vi "Set Stage Speed.vi"(8 "error in (no error)":errorcluster, 9 "Y Axis":u16, 10 "X Axis":u16, 11 "2-Axis Stage in":refnum<class "XY Stage Controller.lvclass">) -> (0 "error out":errorcluster, 3 "2-Axis Stage out":refnum<class "XY Stage Controller.lvclass">)   [LabVIEW 2022 SP3, in "XY Stage Controller.lvclass"]
uses:
  XY Stage Controller.lvclass
  XY Stage Process/XY Stage Process/XY Stage Process Messages/Set Stage Speed Msg/Set Stage Speed Msg.lvclass
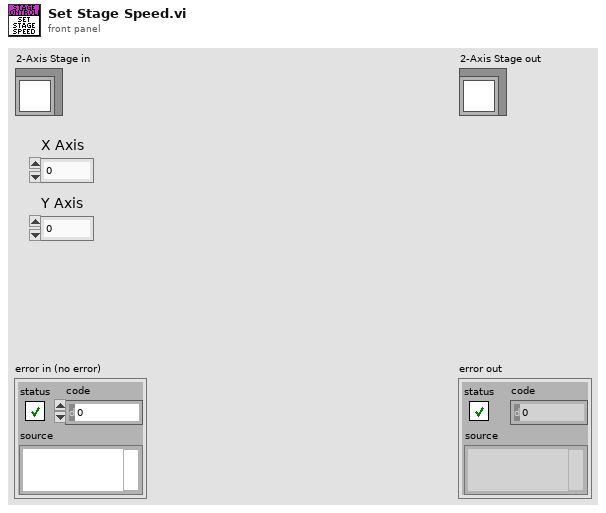
[diagram p1: front panel]
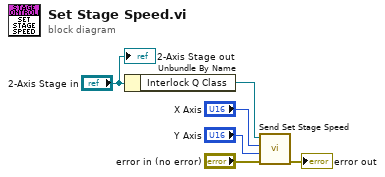
[diagram p0: block diagram]
diagram:
  n1 = Unbundle By Name("2-Axis Stage in") -> ("Interlock Q Class"=w5:refnum<class "Interlock Q Class.lvclass">)
  n2 = call "Send Set Stage Speed.vi"("error in (no error)"="error in (no error)", "Y Axis"="Y Axis", "X Axis"="X Axis", "Interlock Q Class in"=w5) -> ("error out"=→"error out":errorcluster)  [unwired: 6 in, 1 out]
  "2-Axis Stage out" <- "2-Axis Stage in"
